vi "main_RT.vi"() -> ()   [LabVIEW 2015]
uses:
  <vilib>/FPGAPlugInAG/myRIO-1900/niLvFpga_Open_myRIO-1900.vi
  <vilib>/rvi/interface/common/dynamic/niFpgaDynamicAddResources.vi
  <vilib>/Utility/error.llb/Error Cluster From Error Code.vi
  <vilib>/rvi/errors/niLvFpgaAdjustHostInterfaceError.vi
  <vilib>/rvi/interface/nirviOpenFPGA/nirviOpenFPGA.xnode
  FPGA Bitfiles/main_FPGA.lvbitx
  <vilib>/rvi/interface/nirviReadWriteControl/nirviReadWriteControl.xnode
  NiFpgaLv.dll
  <vilib>/rvi/interface/Simulation/niFpgaSimulationCallBeginRW.vi
panel:
  in  "NS Smart":bool
  in  "NS Priority":bool
  in  "West Sensor":bool
  in  "East Sensor":bool
  in  "South Sensor":bool
  in  "North Sensor":bool
  in  "Invert Physical Buttons?":bool
  in  "NS Extend":bool
  out "NS phy button":bool
  out "EW phy button":bool
  out "NS RT button":bool
  out "EW RT button":bool
  out "EW Accepted":bool
  out "NS Accepted":bool
  in  "Accept Physical Inputs?":bool
  in  "Stop":bool
  in  "Cross (NS)":bool
  in  "Cross (EW)":bool
  in  "Start":bool
  out "R(NS)":bool
  out "G(NS)":bool
  out "Y(NS)":bool
  out "R(EW)":bool
  out "G(EW)":bool
  out "Y(EW)":bool
  out "Time(s)":i16
  in  "PR0":bool
  in  "PR1":bool
  out "Clock Frequency (Hz)":i16
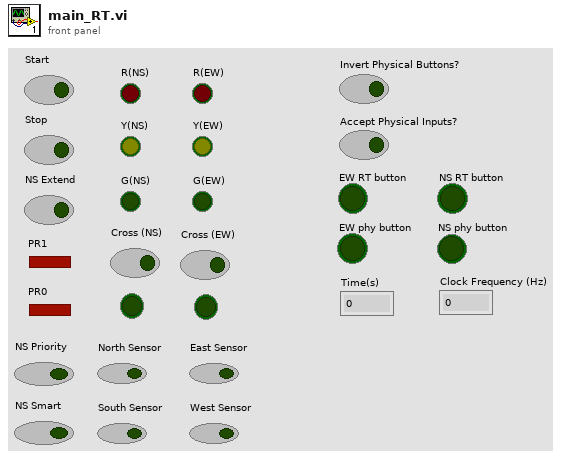
[diagram p1: front panel]
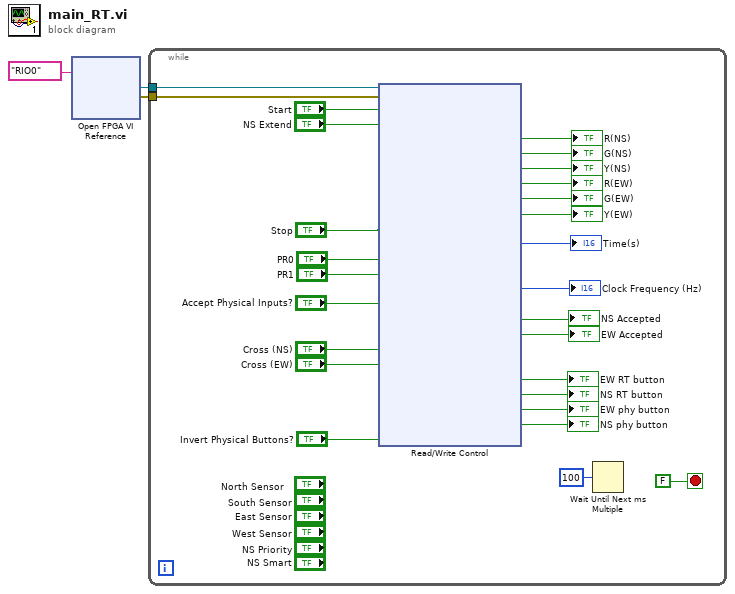
[diagram p0: block diagram]
diagram:
  n1 = xnode "Open FPGA VI Reference"("resource name"=tag "RIO0") -> ("FPGA VI Reference Out"=w2:refnum<k20>, "error out"=w1:errorcluster)  [unwired: 1 in]
  n2 = while {
    tunnel: w2 -> [w30]
    tunnel: w1 -> [w29]
    stop <- FALSE stop-if-true
    n3 = xnode "Read/Write Control"("FPGA VI Reference In"=w30, "error in"=w29, "Start"="Start", "NS Extend"="NS Extend", "Stop"="Stop", "PR0"="PR0", "PR1"="PR1", "Accept Physical Inputs?"="Accept Physical Inputs?", "Crosswalk(EW) new"="Cross (NS)", "Crosswalk(NS) new"="Cross (EW)", "Invert physical buttons"="Invert Physical Buttons?") -> ("R(NS)"=→"R(NS)":bool, "G(NS)"=→"G(NS)":bool, "Y(NS)"=→"Y(NS)":bool, "R(EW)"=→"R(EW)":bool, "G(EW)"=→"G(EW)":bool, "Y(EW)"=→"Y(EW)":bool, "Time(s)"=→"Time(s)":i16, "Clock Frequency (Hz)"=→"Clock Frequency (Hz)":i16, "NS Accepted"=→"NS Accepted":bool, "EW Accepted"=→"EW Accepted":bool, "EW RT button"=→"EW RT button":bool, "NS RT button"=→"NS RT button":bool, "EW phy button"=→"EW phy button":bool, "NS phy button"=→"NS phy button":bool)  [unwired: 2 out]
    n4 = Wait Until Next ms Multiple(millisecond multiple=u32 100) -> ()  [unwired: 1 out]
  }
